vi "Write OCP_Enable.vi"(8 "error in":errorcluster, 10 "OCP_Enable":bool, 11 "SimulatedPS in":refnum<class "SimulatedPS.lvclass">) -> (0 "error out":errorcluster, 3 "SimulatedPS out":refnum<class "SimulatedPS.lvclass">)   [LabVIEW 2019, in "SimulatedPS.lvlib" / "SimulatedPS.lvclass"]
uses:
  Library/SimulatedPS.lvclass
  builds/Instruments/PowerSupply.lvlibp/Library/PowerSupply.lvclass
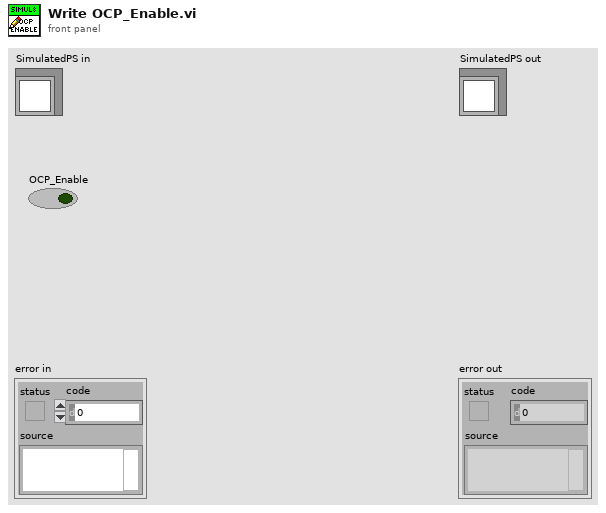
[diagram p1: front panel]
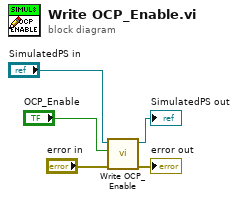
[diagram p0: block diagram]
diagram:
  n1 = call-parent "Write OCP_Enable.vi"("error in"="error in", "OCP_Enable"="OCP_Enable", "PowerSupply in"="SimulatedPS in") -> ("error out"=→"error out":errorcluster, "PowerSupply out"=→"SimulatedPS out":refnum<class "SimulatedPS.lvclass">)  [unwired: 7 in]
